vi "MongoDB.DocumentFind.vi"(8 "error in (no error)":errorcluster, 10 "value":string="{\"test\" : 1}", 11 "MongoDB.Collection in":refnum<class "MongoDB.Collection.lvclass">) -> (0 "error out":errorcluster, 2 "Results Array":string[](array[string]), 3 "MongoDB.Collection out":refnum<class "MongoDB.Collection.lvclass">)   [LabVIEW 2014, in "MongoDB.Collection.lvclass"]
uses:
  MongoDB.Collection.lvclass
  MongoDB.Collection.lvclass/MongoDB.Collection.ctl
  C:/Users/Richard/Documents/GitHub/mongo-labview-driver/CSharp/bin/MongoDB.Driver.Legacy.dll
  CSharp/bin/MongoDB.Driver.Legacy.dll
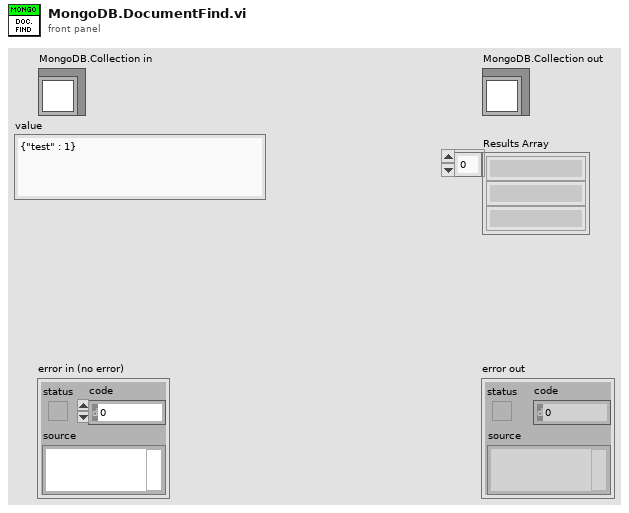
[diagram p1: front panel]
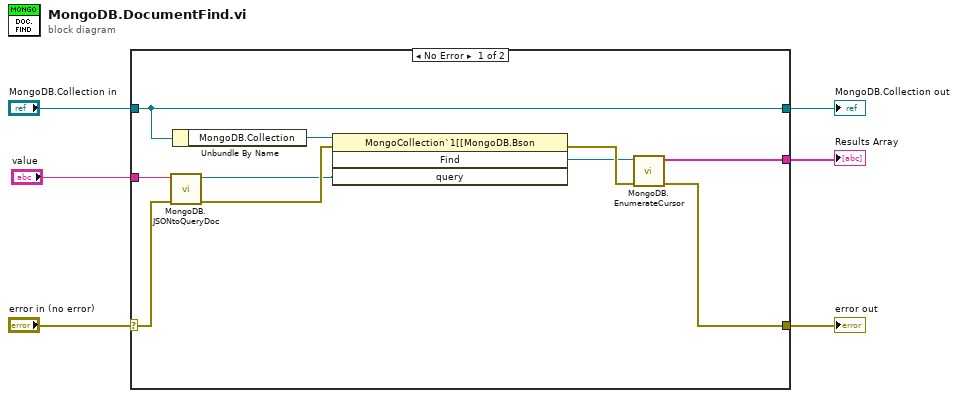
[diagram p0: block diagram]
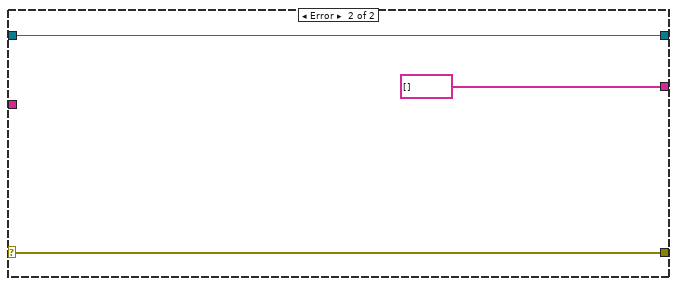
[diagram p2: hidden frame]
diagram:
  n1 = case shown="No Error" "error in (no error)" {
    selector: "error in (no error)" -> [w14 w19]
    tunnel: [w9 w19] -> w5
    tunnel: [w16 w18] -> w3
    tunnel: "MongoDB.Collection in" -> [w16 w18]
    tunnel: "value" -> [w12 _]
    tunnel: [w10 string[] []] -> w1
    frame No Error {
      n2 = call "MongoDB.JSONtoQueryDoc.vi"("error in (no error)"=w14, "JSON Query String"=w12) -> ("error out"=w13:errorcluster, ".NET Refnum out"=w8:refnum<k24>)  [unwired: 8 in]
      n3 = Unbundle By Name(w16) -> ("MongoDB.Collection"=w15:refnum<k24>)
      n4 = invoke class="MongoCollection`1[[MongoDB.Bson" method="Find"(reference=w15, error in=w13, "query"=w8) -> (error out=w11:errorcluster, "Find"=w7:refnum<k24>)  [unwired: 1 in, 2 out]
      n5 = call "MongoDB.EnumerateCursor.vi"("error in (no error)"=w11, "MongoDB.Cursor"=w7) -> ("error out"=w9:errorcluster, "Array"=w10:string[])  [unwired: 8 in]
    }
    frame Error {
    }
  }
  "error out" <- w5
  "MongoDB.Collection out" <- w3
  "Results Array" <- w1
